vi "Tenney Calculate Setpoint.vi"(6 "Humidity Average":dbl, 8 "error in (no error)":errorcluster, 9 "Tenney Environmental Chamber Data Input":T1, 10 "Temperature Limits":T2={"Target Temperature Upper limit"=68.0, "Target Temperature Lower limit"=67.0, "Target Humidity Lower limit"=48.5, "Target Humidity Upper limit"=51.5, "Chamber Temperature Upper limit"=73.0, "Chamber Temperature Lower limit"=63.0, "Chamber Humidity Lower limit"=40.0, "Chamber Humidity Upper limit"=60.0, "Chamber Adjustment Increment (F)"=0.1, "Chamber Adjustment Interval (Minutes)"=10.0, "Chamber Adjustment Increment (%)"=0.1, "Chamber Adjustment Interval Fast (Minutes)"=5.0}, 11 "Temperature Average":dbl) -> (0 "error out":errorcluster, 1 "Tenney Environmental Chamber Data Output":T1, 2 "Humidity In Range?":bool, 3 "Temperature In Range?":bool)   [LabVIEW 2023]
uses:
  controls/Tenney Temperature Limits.ctl
  Drivers/Tidal Engineering/Type Definitions/Tenney Environmental Chamber Data.ctl
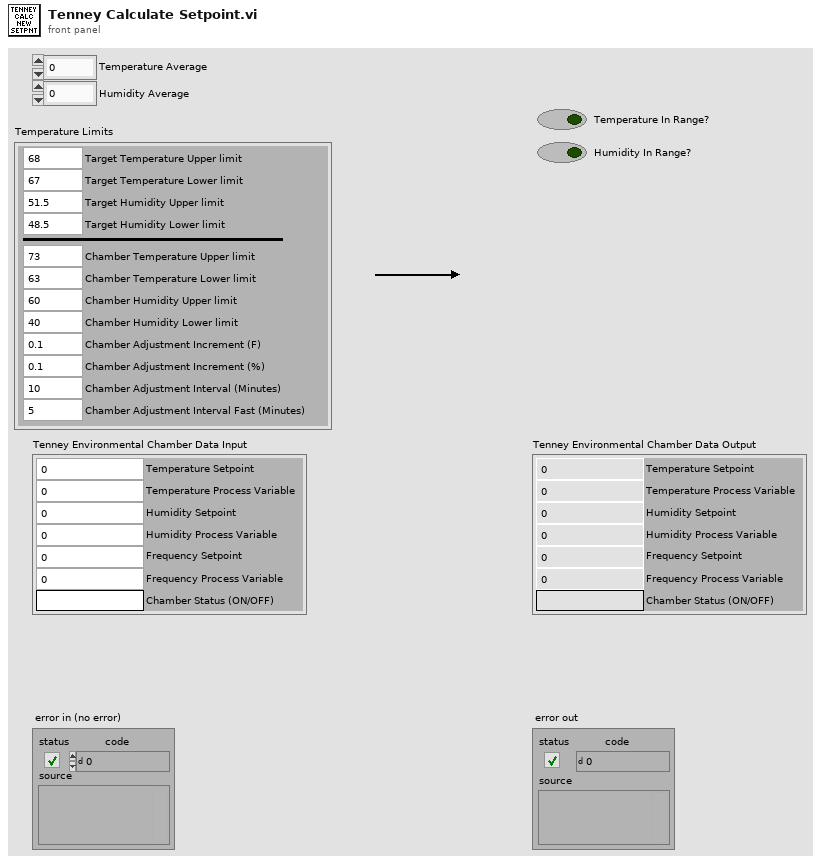
[diagram p1: front panel]
types:
  T1 = typedef "Tenney Environmental Chamber Data.ctl" = cluster{"Temperature Setpoint":dbl, "Temperature Process Variable":dbl, "Humidity Setpoint":dbl, "Humidity Process Variable":dbl, "Frequency Setpoint":dbl, "Frequency Process Variable":dbl, "Chamber Status (ON/OFF)":string}
  T2 = typedef "Tenney Temperature Limits.ctl" = cluster{"Target Temperature Upper limit":dbl, "Target Temperature Lower limit":dbl, "Target Humidity Lower limit":dbl, "Target Humidity Upper limit":dbl, "Chamber Temperature Upper limit":dbl, "Chamber Temperature Lower limit":dbl, "Chamber Humidity Lower limit":dbl, "Chamber Humidity Upper limit":dbl, "Chamber Adjustment Increment (F)":dbl, "Chamber Adjustment Interval (Minutes)":dbl, "Chamber Adjustment Increment (%)":dbl, "Chamber Adjustment Interval Fast (Minutes)":dbl}
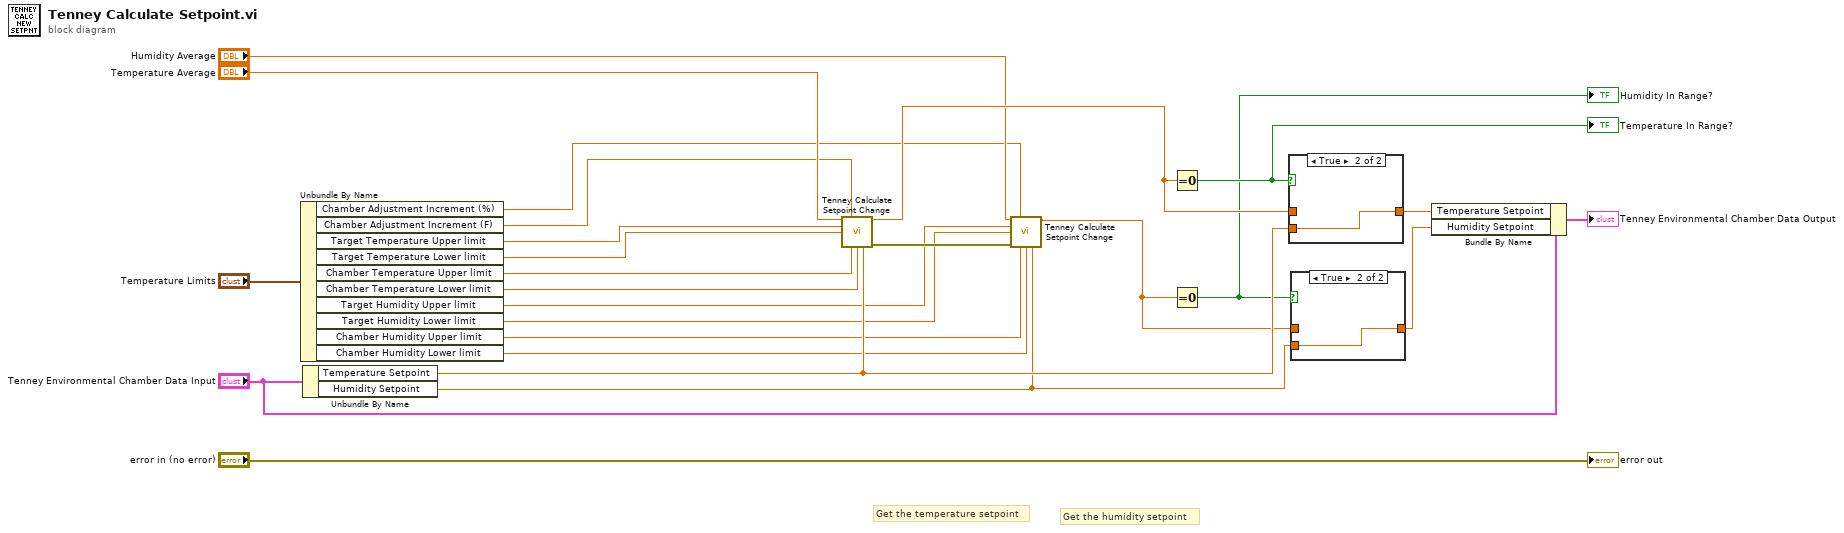
[diagram p0: block diagram]
diagram:
  # "Get the humidity setpoint"
  # "Get the temperature setpoint"
  n1 = Unbundle By Name("Temperature Limits") -> ("Chamber Adjustment Increment (%)"=w1:dbl, "Chamber Adjustment Increment (F)"=w2:dbl, "Target Temperature Upper limit"=w21:dbl, "Target Temperature Lower limit"=w22:dbl, "Chamber Temperature Upper limit"=w18:dbl, "Chamber Temperature Lower limit"=w17:dbl, "Target Humidity Upper limit"=w13:dbl, "Target Humidity Lower limit"=w12:dbl, "Chamber Humidity Upper limit"=w11:dbl, "Chamber Humidity Lower limit"=w10:dbl)
  n2 = Unbundle By Name("Tenney Environmental Chamber Data Input") -> ("Temperature Setpoint"=w16:dbl, "Humidity Setpoint"=w5:dbl)
  n3 = call "Tenney Calculate Setpoint Change.vi"("Average"="Temperature Average", "Adjustment Amount"=w2, "Target Upper limit"=w21, "Target Lower limit"=w22, "Chamber Upper limit"=w18, "Chamber Lower limit"=w17, "Chamber Setpoint"=w16) -> ("new_setpoint"=w19:dbl, "error out"=w15:errorcluster)  [unwired: 7 in]
  n4 = call "Tenney Calculate Setpoint Change.vi"("Average"="Humidity Average", "Adjustment Amount"=w1, "Target Upper limit"=w13, "Target Lower limit"=w12, "error in (no error)"=w15, "Chamber Upper limit"=w11, "Chamber Lower limit"=w10, "Chamber Setpoint"=w5) -> ("new_setpoint"=w6:dbl)  [unwired: 6 in, 1 out]
  n5 = Equal To 0?(x=w19) -> (x = 0?=w20:bool)
  "Temperature In Range?" <- w20
  n6 = Equal To 0?(x=w6) -> (x = 0?=w3:bool)
  "Humidity In Range?" <- w3
  n7 = case shown="True" w20 {
    tunnel: w16 -> [_ w27]
    tunnel: [w26 w27] -> w8
    tunnel: w19 -> [w26 _]
    frame False {
    }
    frame True {
    }
  }
  n8 = case shown="True" w3 {
    tunnel: w5 -> [_ w29]
    tunnel: [w28 w29] -> w4
    tunnel: w6 -> [w28 _]
    frame False {
    }
    frame True {
    }
  }
  n9 = Bundle By Name(cluster="Tenney Environmental Chamber Data Input", "Temperature Setpoint"=w8, "Humidity Setpoint"=w4) -> (→"Tenney Environmental Chamber Data Output":T1)
  "error out" <- "error in (no error)"
